vi "水中油_所有参数读取.vi"(8 "error in (no error)":errorcluster caption="错误输入（无错误）", 11 "MB session in":refnum<class "MB_Master.lvclass">) -> (0 "error out":errorcluster caption="错误输出", 2 "输出值":T1 {"电极型号标志" items=["NULL"=0, "pH"=1, "Cond"=2, "DO"=3, "Turb"=4, "OIW"=17]; "电极状态标志" items=["OK"=0, "第一点校正通过"=1, "第二点校正通过"=2, "悬浮物两点校准第一点校正通过"=11, "悬浮物两点校准第二点校正通过"=12, "浊度三点校正第一点校正通过"=31, "浊度三点校正第二点校正通过"=32, "浊度三点校正第三点校正通过"=33]}, 3 "MB session out":refnum<class "MB_Master.lvclass">)   [LabVIEW 2016, in "斯坦道多参数.lvlib"]
uses:
  <vilib>/Plasmionique/MB Master/MB_Master/MB_Master.lvclass
  <vilib>/Plasmionique/MB Master/MB Master.lvlib
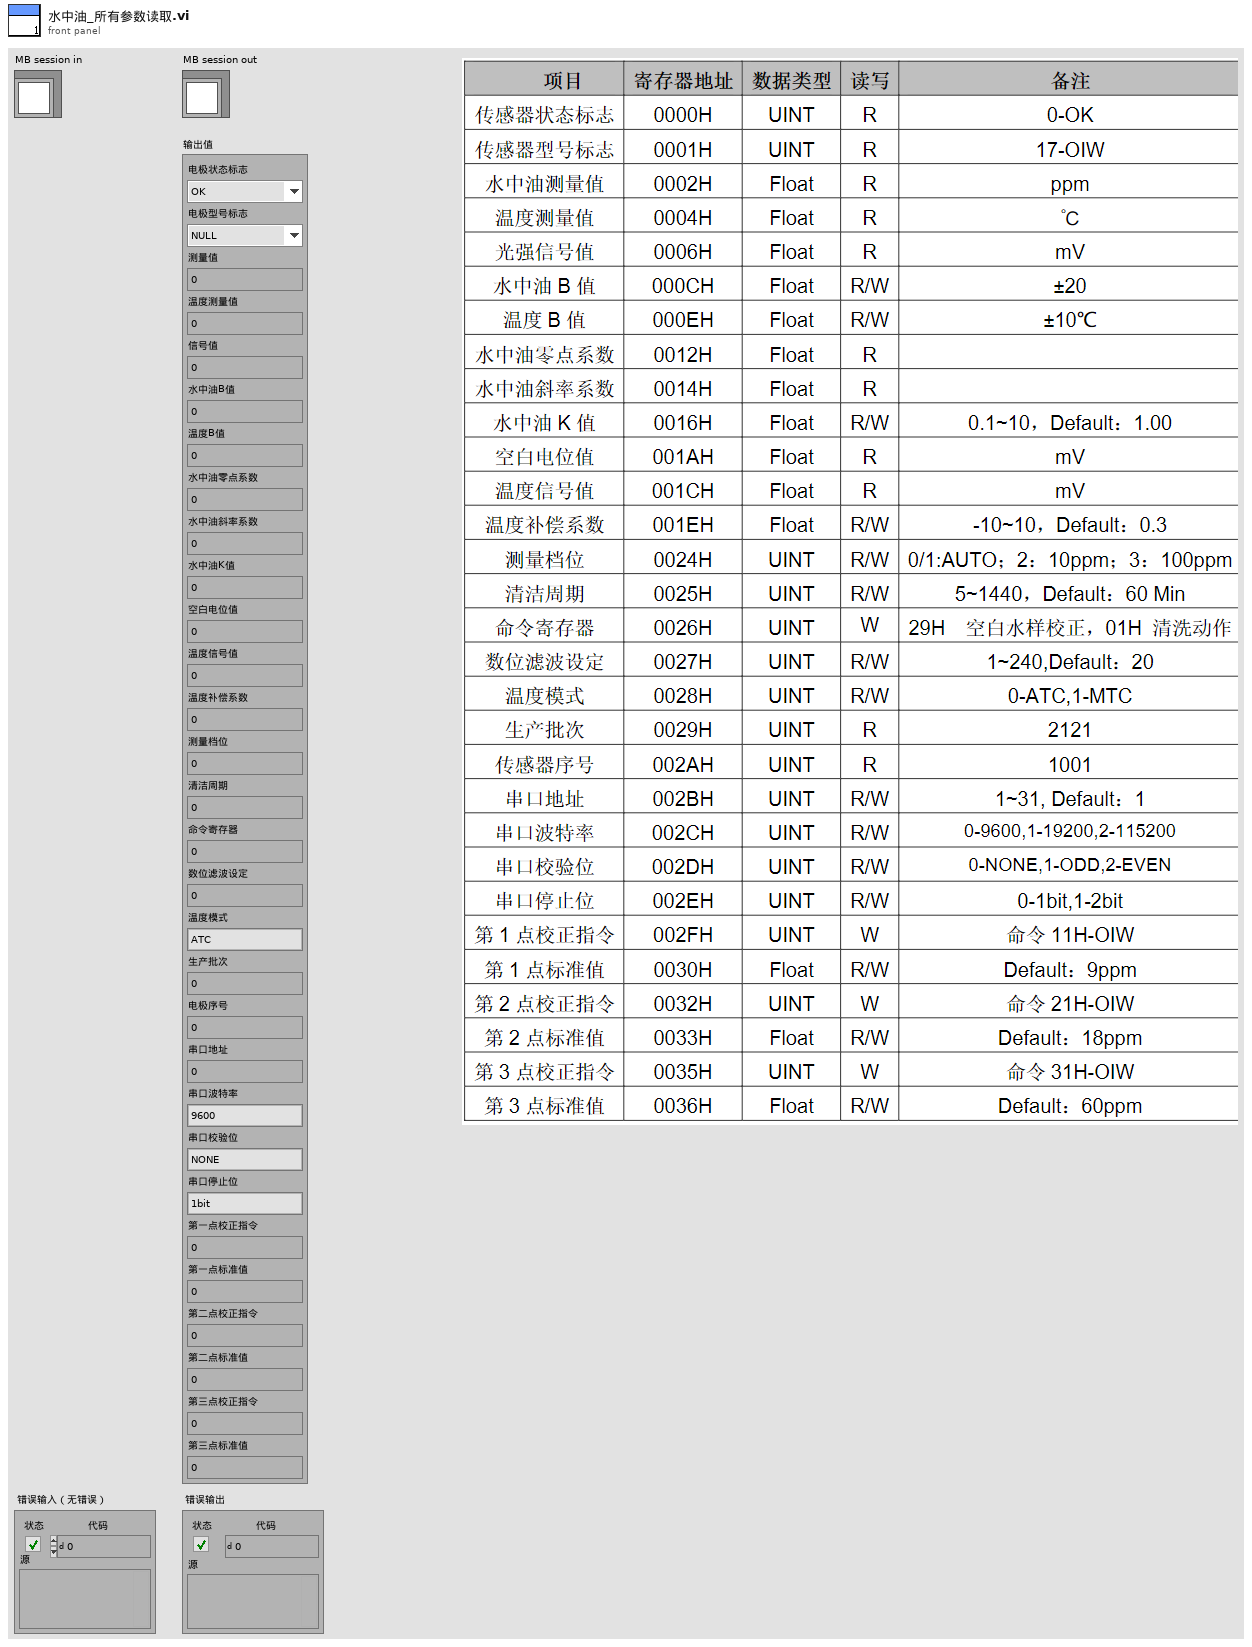
[diagram p1: front panel]
types:
  T1 = cluster{"电极状态标志":u16, "电极型号标志":u16, "测量值":sgl, "温度测量值":sgl, "信号值":sgl, "水中油B值":sgl, "温度B值":sgl, "水中油零点系数":sgl, "水中油斜率系数":sgl, "水中油K值":sgl, "空白电位值":sgl, "温度信号值":sgl, "温度补偿系数":sgl, "测量档位":u16, "清洁周期":u16, "命令寄存器":u16, "数位滤波设定":u16, "温度模式":enum16{"ATC", "MTC"}, "生产批次":u16, "电极序号":u16, "串口地址":u16, "串口波特率":enum16{"9600", "19200", "115200"}, "串口校验位":enum16{"NONE", "ODD", "EVEN"}, "串口停止位":enum16{"1bit", "2bit"}, "第一点校正指令":u16, "第一点标准值":sgl, "第二点校正指令":u16, "第二点标准值":sgl, "第三点校正指令":u16, "第三点标准值":sgl}
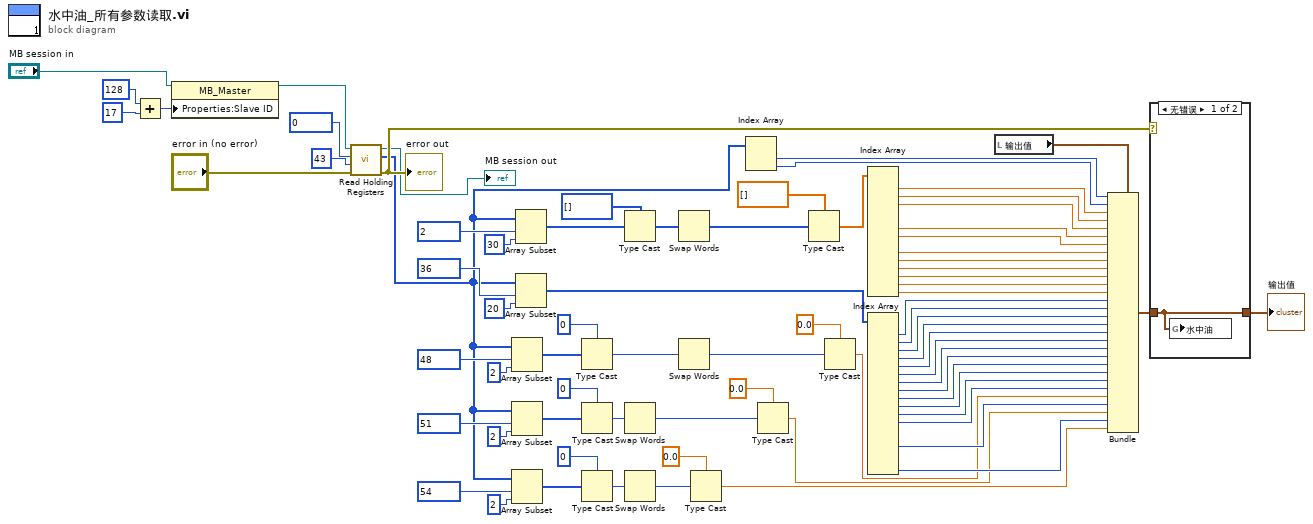
[diagram p0: block diagram]
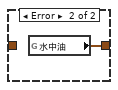
[diagram p2: hidden frame]
diagram:
  n1 = Add(x=u16 128, y=u16 17) -> (x+y=w76:u16)
  n2 = property class="MB_Master"(reference="MB session in", "Properties:Slave ID"=w76) -> (reference out=w42:refnum<class "MB_Master.lvclass">)  [unwired: 1 in, 1 out]
  n3 = call <vilib>:"Read Holding Registers.vi"("error in (no error)"="error in (no error)", "quantity"=u16 43, "starting address"=u16 0, "MB session in"=w42) -> ("error out"=w41:errorcluster, "Registers"=w29:u16[], "MB session out"=→"MB session out":refnum<class "MB_Master.lvclass">)  [unwired: 5 in]
  "error out" <- w41
  n4 = Array Subset(array=w29, index=u16 48 ("starting address"), length=2 ("长度")) -> (w49:u16[])
  n5 = Array Subset(array=w29, index=u16 51 ("starting address"), length=2 ("长度")) -> (w44:u16[])
  n6 = Array Subset(array=w29, index=u16 54 ("starting address"), length=2 ("长度")) -> (w40:u16[])
  n7 = Array Subset(array=w29, index=u16 2 ("starting address"), length=30 ("长度")) -> (w65:u16[])
  n8 = Array Subset(array=w29, index=u16 36 ("starting address"), length=20 ("长度")) -> (w58:u16[])
  n9 = Type Cast(type=u32 0 ("数值"), x=w49) -> (*(type *) &x=w52:u32)
  n10 = Type Cast(type=u32 0 ("数值"), x=w44) -> (*(type *) &x=w46:u32)
  n11 = Type Cast(type=u32 0 ("数值"), x=w40) -> (*(type *) &x=w38:u32)
  n12 = Type Cast(type=u32[] [] ("数组 2"), x=w65) -> (*(type *) &x=w67:u32[])
  n13 = Swap Words(1:w46) -> (0:w45:u32)
  n14 = Swap Words(1:w38) -> (0:w39:u32)
  n15 = Swap Words(1:w67) -> (0:w69:u32[])
  n16 = Swap Words(1:w52) -> (0:w53:u32)
  n17 = Type Cast(type=sgl 0.0 ("数值"), x=w39) -> (*(type *) &x=w2:sgl)
  n18 = Index Array(array=w29) -> (element #1=w72:u16, element #2=w71:u16)  [unwired: 2 in]
  n19 = Type Cast(type=sgl 0.0 ("数值"), x=w45) -> (*(type *) &x=w3:sgl)
  n20 = Type Cast(type=sgl[] [] ("数组 2"), x=w69) -> (*(type *) &x=w64:sgl[])
  n21 = Type Cast(type=sgl 0.0 ("数值"), x=w53) -> (*(type *) &x=w4:sgl)
  n22 = Index Array(array=w64) -> (element #1=w31:sgl, element #2=w63:sgl, element #3=w62:sgl, element #6=w27:sgl, element #7=w26:sgl, element #9=w1:sgl, element #10=w25:sgl, element #11=w24:sgl, element #12=w23:sgl, element #13=w22:sgl, element #14=w21:sgl)  [unwired: 14 in, 3 out]
  n23 = Index Array(array=w58) -> (element #1=w18:u16, element #2=w17:u16, element #3=w16:u16, element #4=w15:u16, element #5=w14:u16, element #6=w13:u16, element #7=w12:u16, element #8=w11:u16, element #9=w10:u16, element #10=w9:u16, element #11=w8:u16, element #12=w7:u16, element #15=w6:u16, element #18=w5:u16)  [unwired: 18 in, 4 out]
  n24 = local read "输出值"() -> (w19:T1)
  n25 = Bundle(cluster=w19, "电极状态标志"=w72, "电极型号标志"=w71, "测量值"=w31, "温度测量值"=w63, "信号值"=w62, "水中油B值"=w27, "温度B值"=w26, "水中油零点系数"=w1, "水中油斜率系数"=w25, "水中油K值"=w24, "空白电位值"=w23, "温度信号值"=w22, "温度补偿系数"=w21, "测量档位"=w18, "清洁周期"=w17, "命令寄存器"=w16, "数位滤波设定"=w15, "温度模式"=w14, "生产批次"=w13, "电极序号"=w12, "串口地址"=w11, "串口波特率"=w10, "串口校验位"=w9, "串口停止位"=w8, "第一点校正指令"=w7, "第一点标准值"=w4, "第二点校正指令"=w6, "第二点标准值"=w3, "第三点校正指令"=w5, "第三点标准值"=w2) -> (w20:T1)
  n26 = case shown="无错误" w41 {
    tunnel: [w77 w78] -> w30
    tunnel: w20 -> [w77 _]
    frame No Error {
      n27 = global write "国弘过程全局变量.vi" "水中油"(w77) -> ()
    }
    frame Error {
      n28 = global read "国弘过程全局变量.vi" "水中油"() -> (w78:T1)
    }
  }
  "输出值" <- w30
